vi "Static References, Strictly or not Strictly Typed.vi"   [LabVIEW 2020]
panel:
  # "Broken code, just for illustration.\nSee diagram."
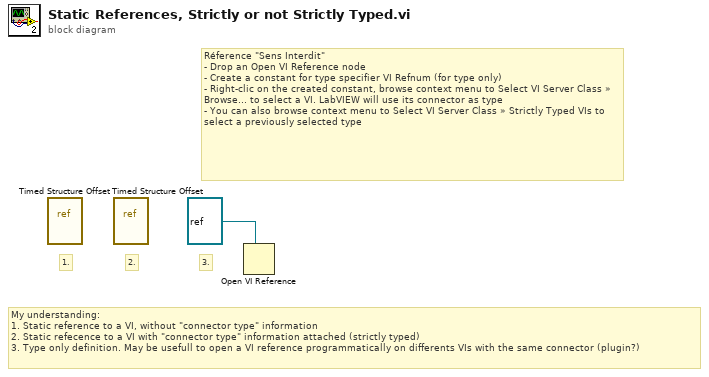
[diagram p0: block diagram]
diagram:
  # "3."
  # "2."
  # "1."
  # "My understanding:\n1. Static reference to a VI, without \"connector type\" information\n2. Static refecence to a VI with \"connector type\" information attached (strictly typed)\n3. Type only definition. May be usefull to open a VI reference programmatically on differents VIs with the same connector (plugin?)"
  # "Réference \"Sens Interdit\"\n- Drop an Open VI Reference node\n- Create a constant for type specifier VI Refnum (for type only)\n- Right-clic on the created constant, browse context menu to Select VI Server Class » Browse... to select a VI. LabVIEW will use its connector as type\n- You can also browse context menu to Select VI Server Class » Strictly Typed VIs to select a previously selected type"
  n1 = vi-ref "Timed Structure Offset.vi"() -> ()  [unwired: 1 out]
  n2 = vi-ref "Timed Structure Offset.vi"() -> ()  [unwired: 1 out]
  n3 = Open VI Reference(type specifier VI Refnum (for type only)=refnum<vi> refnum) -> ()  [unwired: 5 in, 2 out]
